vi "range.vi"(10 "x0":i32, 11 "N":i32) -> (2 "Range":i32[](array[numeric]))   [LabVIEW 2020]
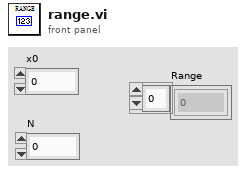
[diagram p1: front panel]
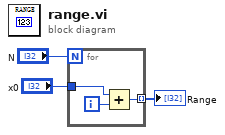
[diagram p0: block diagram]
diagram:
  n1 = for {
    N: "N" -> [_]
    tunnel: [w6] -> w2 mode=indexing
    tunnel: "x0" -> [w5]
    i -> [w4]
    n2 = Add(x=w5, y=w4) -> (x+y=w6:i32)
  }
  "Range" <- w2
